vi "c Spark Get API Version.vi"(8 "error in (no error)":errorcluster) -> (0 "error out":errorcluster, 2 "c_Spark_APIVersion":T1, 3 "function return":u64)   [LabVIEW 2023, in "REVLibDriver.lvlib"]
doc: "c_Spark_APIVersion c_Spark_GetAPIVersion(void);"
uses:
  REVLibDriver.lvlib
  REVLibDriver.dll
  Custom Controls/c_Spark_APIVersion.ctl
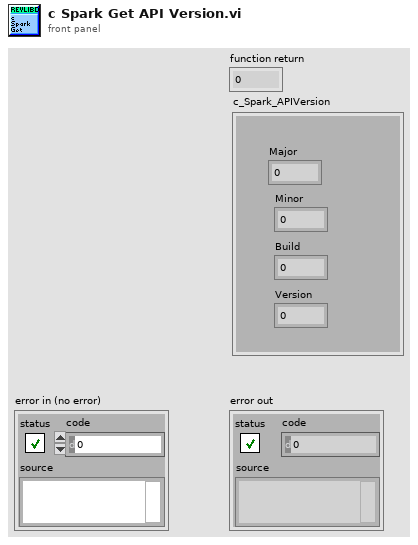
[diagram p1: front panel]
types:
  T1 = typedef "REVLibDriver.lvlib/c_Spark_APIVersion.ctl" = cluster{"Major":u16, "Minor":u8, "Build":u8, "Version":u32}
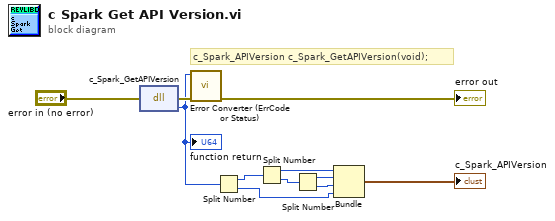
[diagram p0: block diagram]
diagram:
  # "c_Spark_APIVersion c_Spark_GetAPIVersion(void);"
  n1 = dll-call lib="REVLibDriver.*" fn="c_Spark_GetAPIVersion"(error in="error in (no error)") -> (error out=w10:errorcluster, "return type"=w2:u64)  [unwired: 2 in, 1 out]
  "function return" <- w2
  n2 = call "Error Converter (ErrCode or Status).vi"("error in (no error)"=w10, "error code"=w2) -> ("error out"=→"error out":errorcluster)  [unwired: 9 in]
  n3 = Split Number(x=w2) -> (hi(x)=w8:u32, lo(x)=w3:u32)
  n4 = Split Number(x=w8) -> (hi(x)=w6:u16, lo(x)=w7:u16)
  n5 = Split Number(x=w7) -> (hi(x)=w5:u8, lo(x)=w4:u8)
  n6 = Bundle(w6, w5, w4, w3) -> (→"c_Spark_APIVersion":cluster{u16, u8, u8, u32})  [unwired: 1 in]
